vi "Prepare Response.vi"(8 "error in (no error)":errorcluster, 10 "Request":refnum<class "Request.lvclass">) -> (0 "error out":errorcluster, 2 "Response":refnum<class "Response.lvclass">, 5 "Last Event ID":string)   [LabVIEW 2020, in "HTTP Server.lvlib" / "SSE Handler.lvclass"]
uses:
  SSE Handler.lvclass
  SSE Handler.lvclass/SSE Handler.ctl
  lv-http-util/HTTP Utils/Response/Response.lvclass
  lv-http-util/HTTP Utils/Request/Request.lvclass
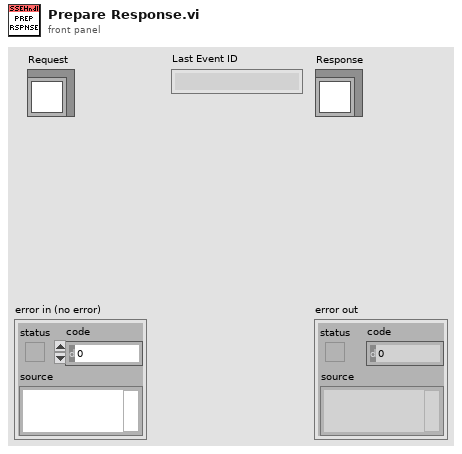
[diagram p1: front panel]
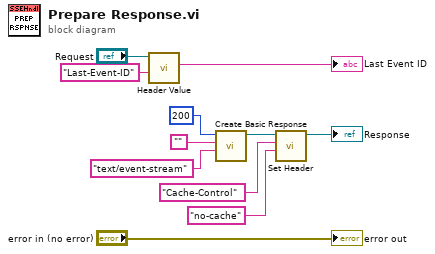
[diagram p0: block diagram]
diagram:
  n1 = call "Header Value.vi"("Header"="Last-Event-ID", "Request in"="Request") -> ("Value"=→"Last Event ID":string)  [unwired: 6 in, 3 out]
  n2 = call "Create Basic Response.vi"("Content-Type (text/plain)"="text/event-stream", "Payload"="", "Status Code"=u16 200) -> ("Response out"=w8:refnum<class "Response.lvclass">)  [unwired: 7 in, 1 out]
  n3 = call "Set Header.vi"("Value"="no-cache" ("Content-Type (text/plain)"), "Header"="Cache-Control" ("Content-Type (text/plain)"), "Response in"=w8) -> ("Response out"=→"Response":refnum<class "Response.lvclass">)  [unwired: 6 in, 2 out]
  "error out" <- "error in (no error)"
